vi "TraverseControl_High.vi"(0 "Mode":T3=enum."Read traverse position", 1 "Route Checking?":bool, 2 "Home":T2, 3 "Traverse Name":string, 5 "Extra command String":string, 6 "Work in Tunnel Coordinates":T1, 7 "Model       Roll      Pitch       Yaw (deg)":sgl[](array[numeric]) format="%#.2f", 9 "Final iteration of 3D_Trav Loop":bool=TRUE, 11 "Position input XYZ Always Tunnel":sgl[](array[numeric])=[0.0, 0.0, 0.0] format="%.2f", 12 "Last Part of Move?":bool, 13 "Speed Factor":sgl=1.0 min=0.1 max=5 format="%.2f", 14 "Backlash Compensation?":bool=TRUE) -> (4 "Position Output XYZ":sgl[](array[numeric]) format="%.2f", 10 "Position Correct":bool, 15 "Error String":string)   [LabVIEW 2022 SP3]
uses:
  Anemometry/Anemometry Sub Vis/Gen Trav/Trav_mode.ctl
  Anemometry/Anemometry Sub Vis/Controls/Home.ctl
  Anemometry/Anemometry Sub Vis/Controls/Tunnel_Coordinates.ctl
  Anemometry/Anemometry Sub Vis/Globals/Extra_Commands_Global.vi
  Anemometry/Anemometry Sub Vis/Globals/Trav_pos_global.vi
  Anemometry/Anemometry Sub Vis/Gen Trav/Route mapping/Route_mapping_global.vi
panel:
  out "Offset Array":sgl[](array[numeric])
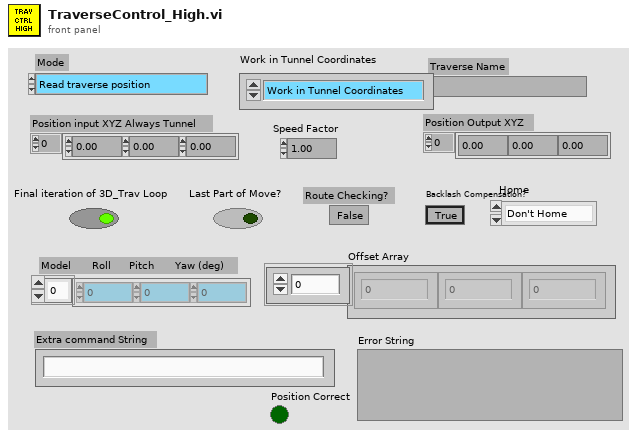
[diagram p1: front panel]
types:
  T1 = typedef "Tunnel_Coordinates.ctl" = enum16{"Work in Tunnel Coordinates", "Work in Model Coordinates"}
  T2 = typedef "Home.ctl" = enum16{"Don't Home", "Home  +X", "Home  -X", "Home  +Y", "Home  -Y", "Home  +Z", "Home  -Z"}
  T3 = typedef "Trav_mode.ctl" = enum16{"Move traverse", "Read traverse position", "Teach Position"}
  T4 = enum16{"To Traverse Coordinates", "To User Coordinates"}
  T5 = typedef "Axis.ctl" = enum16{"X Axis", "X Axis -ve", "Y Axis", "Y Axis -ve", "Z Axis", "Z Axis -ve"}
  T6 = typedef "Box_size.ctl" = cluster{"Max":sgl, "Min":sgl}[]
  T7 = typedef "Exclude_cluster.ctl" = cluster{"Sizes":T6, "Name":string, "Exclude Type":T8}
  T8 = typedef "Exclusion_type.ctl" = enum16{"Exclude completely", "Allow only vertical moves"}
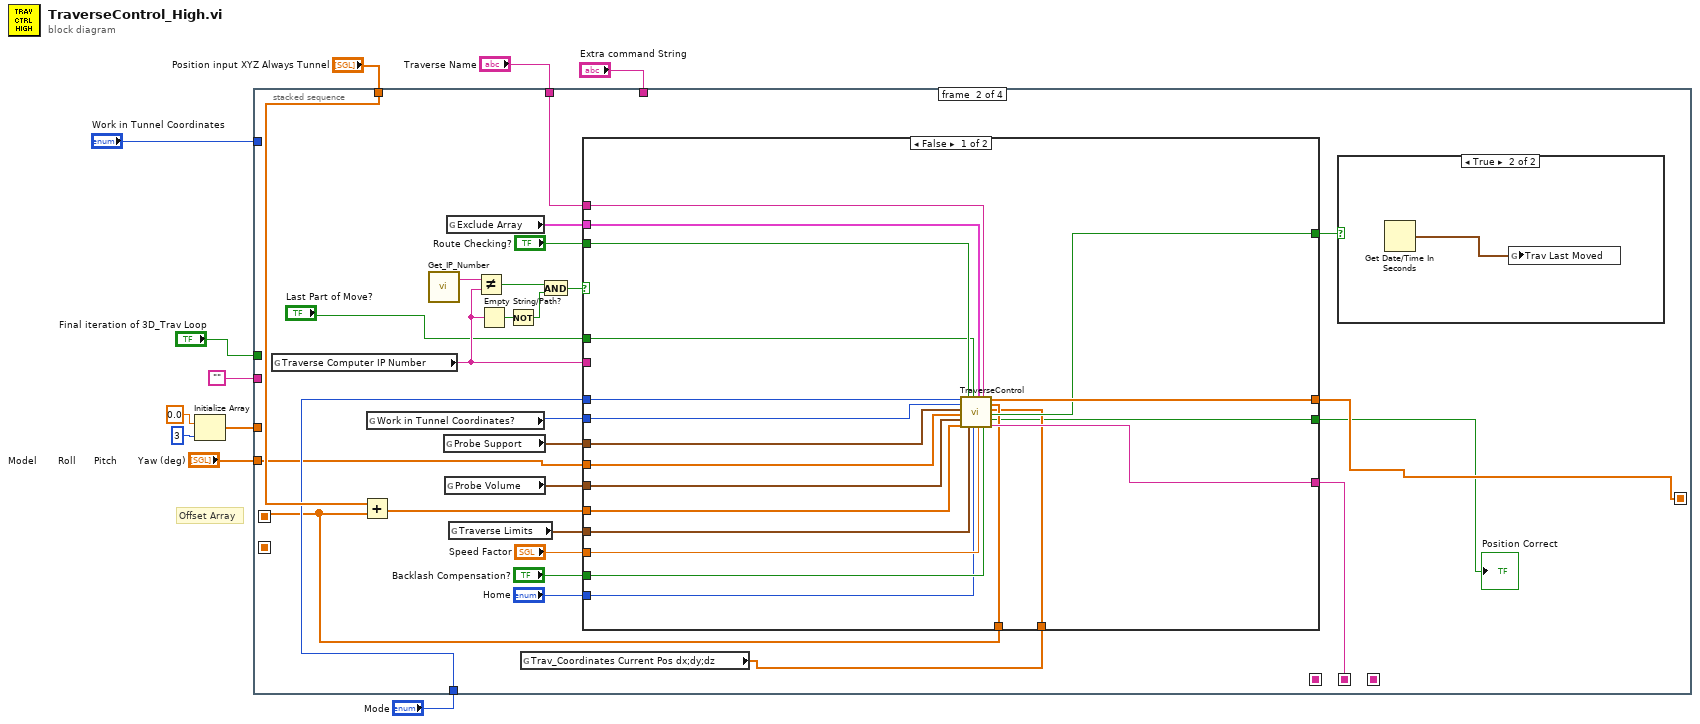
[diagram p0: block diagram]
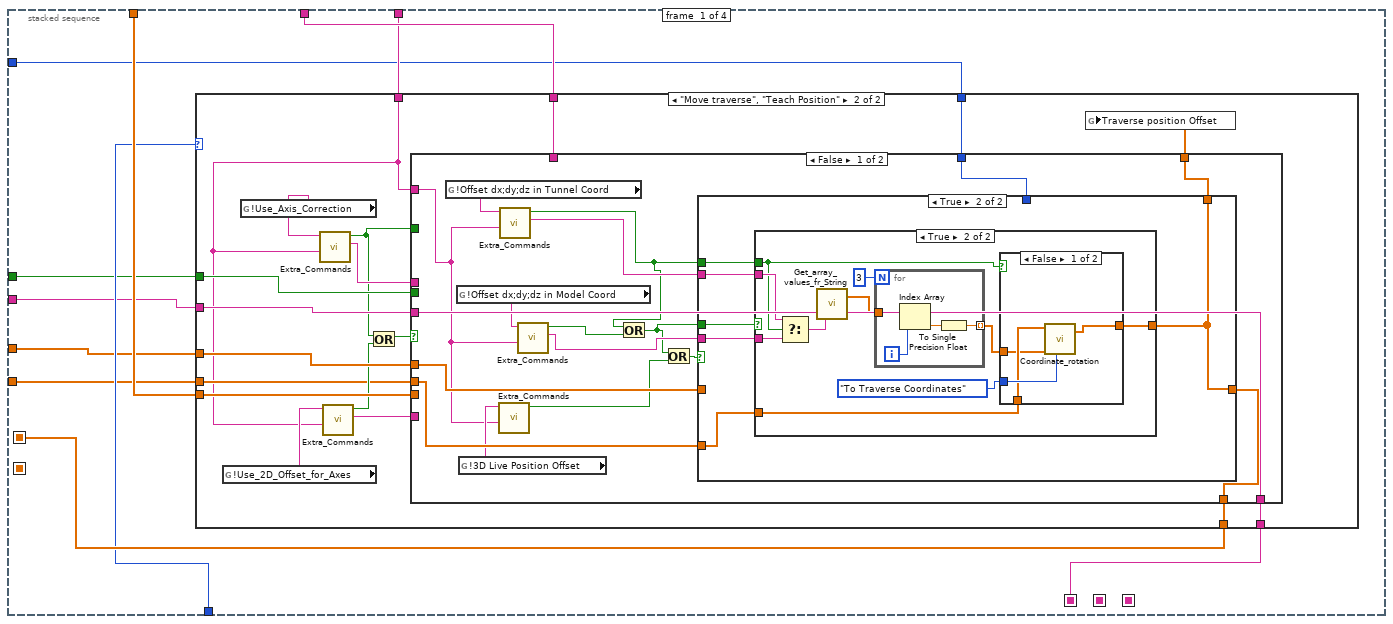
[diagram p2: hidden frame]
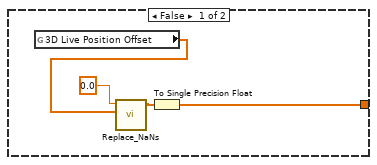
[diagram p5: hidden frame]
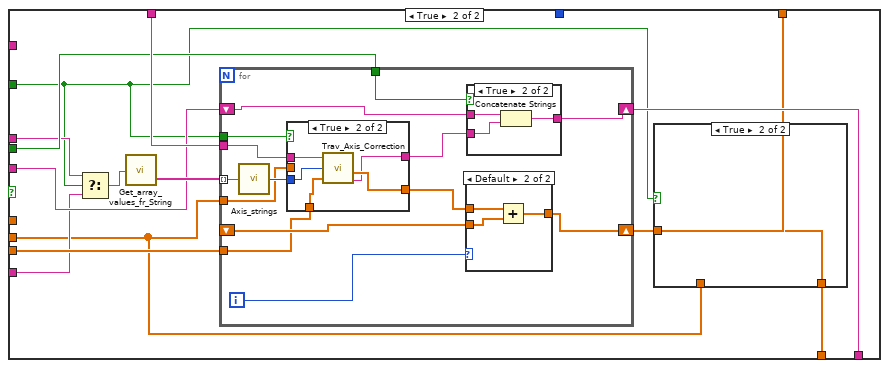
[diagram p7: hidden frame]
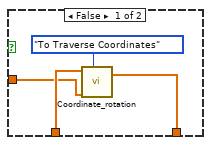
[diagram p8: hidden frame]
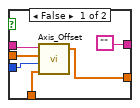
[diagram p9: hidden frame]
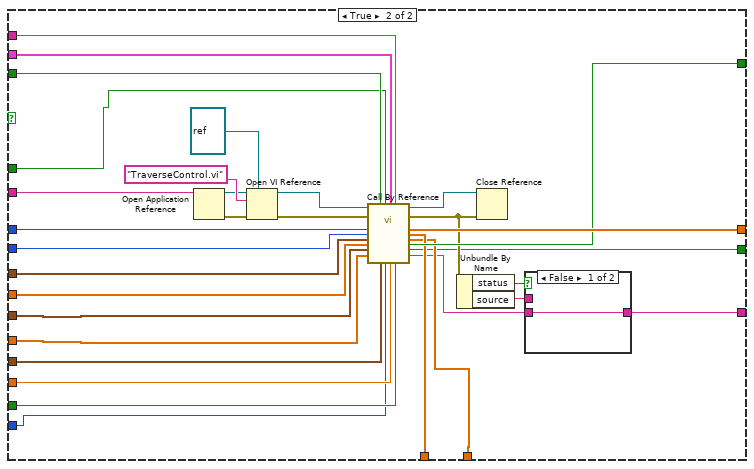
[diagram p13: hidden frame]
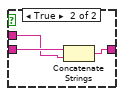
[diagram p14: hidden frame]
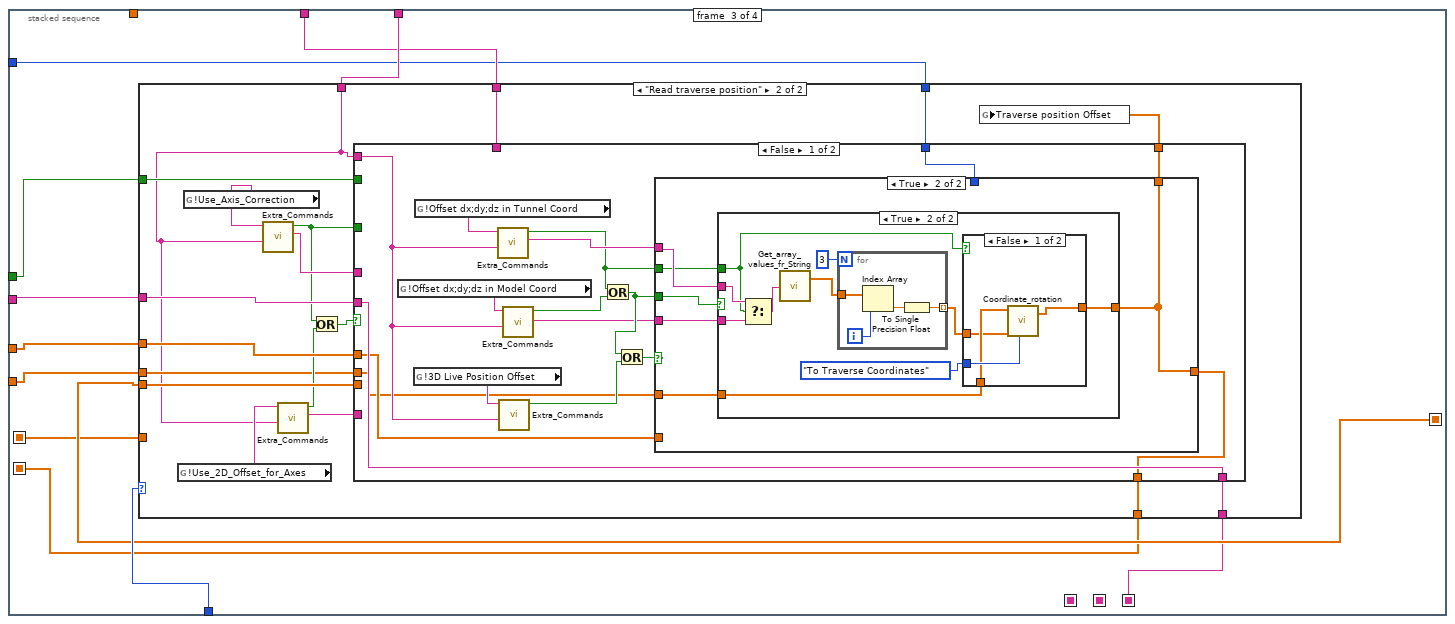
[diagram p15: hidden frame]
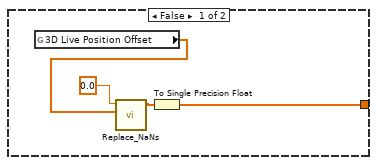
[diagram p18: hidden frame]
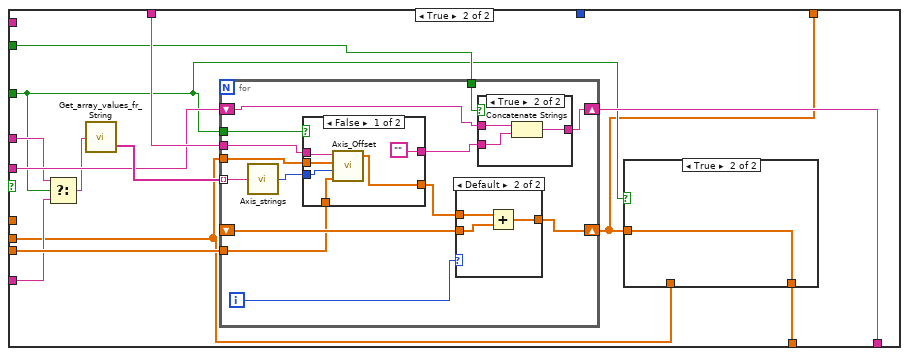
[diagram p20: hidden frame]
diagram:
  # "Offset Array"
  n1 = Initialize Array(sgl 0.0, 3 ("dimension size")) -> (w5:sgl[])
  n2 = stacked-sequence {
    seq-local: [_ w151 _ _] -> [_ _ w232 w360]
    seq-local: [w22 _ _ _] -> [_ w143 w228 _]
    seq-local: [w19 _ _ _] -> [_ _ _ w356]
    seq-local: [_ _ w230 _] -> [_ _ _ w355]
    seq-local: [_ _ w229 _] -> [_ _ _ w358]
    seq-local: [_ w146 _ _] -> [_ _ _ w357]
    tunnel: "Traverse Name" -> [w21 w150 w234 _]
    tunnel: "Position input XYZ Always Tunnel" -> [w20 w149 _ _]
    tunnel: "Mode" -> [w17 w147 w236 _]
    tunnel: "Extra command String" -> [w18 _ w235 _]
    tunnel: w5 -> [w16 _ w231 _]
    tunnel: "" -> [w15 _ w233 _]
    tunnel: "Final iteration of 3D_Trav Loop" -> [w14 _ w227 _]
    tunnel: "Model       Roll      Pitch       Yaw (deg)" -> [w13 w144 w226 _]
    tunnel: "Work in Tunnel Coordinates" -> [w12 _ w225 _]
    frame #0 {
      n3 = case shown="\"Move traverse\", \"Teach Position\"" w17 {
        tunnel: [w23 w41] -> w22
        tunnel: w21 -> [_ w40]
        tunnel: w20 -> [_ w38]
        tunnel: [w24 w37] -> w19
        tunnel: w18 -> [_ w27]
        tunnel: w16 -> [w23 w36]
        tunnel: w15 -> [w24 w35]
        tunnel: w14 -> [_ w34]
        tunnel: w13 -> [_ w28]
        tunnel: w12 -> [_ w25]
        frame Default {
        }
        frame "Move traverse", "Teach Position" {
          n4 = global read "Extra_Commands_Global.vi" "!Use_2D_Offset_for_Axes"() -> (w33:string)
          n5 = global read "Extra_Commands_Global.vi" "!Use_Axis_Correction"() -> (w42:string)
          n6 = call "Extra_Commands.vi"("String to Search"=w27, "Command"=w42) -> ("String Value"=w39:string, "Command Found"=w30:bool)  [unwired: 1 in, 3 out]
          n7 = call "Extra_Commands.vi"("String to Search"=w27, "Command"=w33) -> ("String Value"=w29:string, "Command Found"=w32:bool)  [unwired: 1 in, 3 out]
          n8 = Or(x=w30, y=w32) -> (x .or. y?=w31:bool)
          n9 = case shown="False" w31 {
            tunnel: [w55 w92] -> w41
            tunnel: w38 -> [_ w100]
            tunnel: w40 -> [_ w101]
            tunnel: w39 -> [_ w96]
            tunnel: [w59 w97] -> w37
            tunnel: w35 -> [w59 w99]
            tunnel: w36 -> [w56 _]
            tunnel: w34 -> [_ w98]
            tunnel: w30 -> [_ w91]
            tunnel: w29 -> [_ w95]
            tunnel: w28 -> [w53 w93]
            tunnel: w27 -> [w45 _]
            tunnel: [w52 w90] -> w26
            tunnel: w25 -> [w54 _]
            frame False {
              n10 = global read "Extra_Commands_Global.vi" "!Offset dx;dy;dz in Tunnel Coord"() -> (w58:string)
              n11 = global read "Extra_Commands_Global.vi" "!Offset dx;dy;dz in Model Coord"() -> (w46:string)
              n12 = global read "Extra_Commands_Global.vi" "!3D Live Position Offset"() -> (w49:string)
              n13 = call "Extra_Commands.vi"("String to Search"=w45, "Command"=w49) -> ("Command Found"=w51:bool)  [unwired: 1 in, 4 out]
              n14 = call "Extra_Commands.vi"("String to Search"=w45, "Command"=w58) -> ("String Value"=w57:string, "Command Found"=w48:bool)  [unwired: 1 in, 3 out]
              n15 = call "Extra_Commands.vi"("String to Search"=w45, "Command"=w46) -> ("String Value"=w44:string, "Command Found"=w47:bool)  [unwired: 1 in, 3 out]
              n16 = Or(x=w48, y=w47) -> (x .or. y?=w43:bool)
              n17 = Or(x=w43, y=w51) -> (x .or. y?=w50:bool)
              n18 = case shown="True" w50 {
                tunnel: w57 -> [_ w64]
                tunnel: [w60 w66] -> w55
                tunnel: w56 -> [w60 _]
                tunnel: w54 -> [_ _]
                tunnel: w53 -> [_ w65]
                tunnel: [w60 w66] -> w52
                tunnel: w48 -> [_ w61]
                tunnel: w44 -> [_ w63]
                tunnel: w43 -> [_ w62]
                frame False {
                }
                frame True {
                  n19 = case shown="True" w62 {
                    tunnel: [w67 w75] -> w66
                    tunnel: w65 -> [_ w77]
                    tunnel: w64 -> [_ w74]
                    tunnel: w63 -> [_ w73]
                    tunnel: w61 -> [_ w72]
                    frame False {
                      n20 = global read "Trav_pos_global.vi" "3D Live Position Offset"() -> (w69:sgl[])
                      n21 = call "Replace_NaNs.vi"("Array"=w69, "Replacement"=0.0) -> ("Array Out"=w68:dbl[])  [unwired: 9 in]
                      n22 = To Single Precision Float(number=w68) -> (single precision float=w67:sgl[])
                    }
                    frame True {
                      n23 = Select(t=w74, s=w72, f=w73) -> (s? t:f=w71:string)
                      n24 = call "Get_array_values_fr_String.vi"("String Value"=w71) -> ("Numeric Array"=w79:dbl[])  [unwired: 1 out]
                      n25 = for {
                        N: 3 -> [_]
                        tunnel: w79 -> [w89]
                        tunnel: [w86] -> w76 mode=indexing
                        i -> [w88]
                        n26 = Index Array(array=w89, index=w88) -> (element=w87:dbl)
                        n27 = To Single Precision Float(number=w87) -> (single precision float=w86:sgl)
                      }
                      n28 = case shown="False" w72 {
                        tunnel: T4."To Traverse Coordinates" ("Mode") -> [w84 _]
                        tunnel: w77 -> [w83 _]
                        tunnel: w76 -> [w82 w85]
                        tunnel: [w81 w85] -> w75
                        frame False {
                          n29 = call "Coordinate_rotation.vi"("Roll-Pitch-Yaw"=w83, "Input Position"=w82, "Mode"=w84) -> ("Output Position"=w81:sgl[])  [unwired: 2 in, 1 out]
                        }
                        frame True {
                        }
                      }
                    }
                  }
                }
              }
            }
            frame True {
              n30 = Select(t=w96, s=w91, f=w95) -> (s? t:f=w94:string)
              n31 = call "Get_array_values_fr_String.vi"("String Value"=w94) -> ("String array"=w102:string[])  [unwired: 1 out]
              n32 = for {
                tunnel: w102 -> [w121] mode=indexing
                tunnel: w101 -> [w114]
                tunnel: w100 -> [w112]
                shift-right: [w119] -> w90
                shift-left: _ -> [w120]
                shift-right: [w116] -> w97
                shift-left: w99 -> [w117]
                tunnel: w98 -> [w115]
                tunnel: w91 -> [w108]
                tunnel: w93 -> [w109]
                i -> [w118]
                n33 = call "Axis_strings.vi"("String"=w121) -> ("Enum"=w113:T5)
                n34 = case shown="True" w108 {
                  tunnel: w114 -> [w126 w132]
                  tunnel: w113 -> [w125 w131]
                  tunnel: w112 -> [w124 w130]
                  tunnel: [w127 w129] -> w111
                  tunnel: ["" w128] -> w110
                  tunnel: w109 -> [w122 _]
                  frame False {
                    n35 = call "Axis_Offset.vi"("Position In"=w124, "Axis"=w125, "Roll-Pitch-Yaw"=w122, "Traverse Name"=w126) -> ("Offset Array"=w127:sgl[])  [unwired: 2 out]
                  }
                  frame True {
                    n36 = call "Trav_Axis_Correction.vi"("Traverse Name"=w132, "Axis"=w131, "Position input XYZ"=w130) -> ("Offset Array"=w129:sgl[], "Error String"=w128:string)  [unwired: 2 out]
                  }
                }
                n37 = case shown="Default" w118 {
                  tunnel: w111 -> [w137 w140]
                  tunnel: w120 -> [_ w139]
                  tunnel: [w137 w138] -> w119
                  frame 0 {
                  }
                  frame Default {
                    n38 = Add(x=w140, y=w139) -> (x+y=w138:sgl[])
                  }
                }
                n39 = case shown="True" w115 {
                  tunnel: w110 -> [_ w136]
                  tunnel: w117 -> [w133 w135]
                  tunnel: [w133 w134] -> w116
                  frame False {
                  }
                  frame True {
                    n40 = Concatenate Strings(w135, w136) -> (w134:string)
                  }
                }
              }
              n41 = case shown="True" w91 {
                tunnel: w90 -> [w103 w107]
                tunnel: w93 -> [w106 _]
                tunnel: [w105 w107] -> w92
                frame False {
                  n42 = call "Coordinate_rotation.vi"("Roll-Pitch-Yaw"=w106, "Input Position"=w103, "Mode"=T4."To Traverse Coordinates") -> ("Output Position"=w105:sgl[])  [unwired: 2 in, 1 out]
                }
                frame True {
                }
              }
            }
          }
          n43 = global write "Trav_pos_global.vi" "Traverse position Offset"(w26) -> ()
        }
      }
    }
    frame #1 {
      n44 = global read "Trav_pos_global.vi" "Traverse Computer IP Number"() -> (w161:string)
      n45 = Add(x=w149, y=w143) -> (x+y=w148:sgl[])
      n46 = global read "Trav_pos_global.vi" "Work in Tunnel Coordinates?"() -> (w155:T1)
      n47 = call "Get_IP_Number.vi"() -> ("IP Number"=w167:string)  [unwired: 1 out]
      n48 = global read "Route_mapping_global.vi" "Probe Support"() -> (w154:T6)
      n49 = global read "Route_mapping_global.vi" "Probe Volume"() -> (w156:T6)
      n50 = global read "Route_mapping_global.vi" "Exclude Array"() -> (w158:T7[])
      n51 = global read "Route_mapping_global.vi" "Traverse Limits"() -> (w157:T6)
      n52 = Not Equal?(x=w167, y=w161) -> (x != y?=w160:bool)
      n53 = Empty String/Path?(string/path=w161) -> (empty?=w163:bool)
      n54 = Not(x=w163) -> (.not. x?=w162:bool)
      n55 = global read "Trav_pos_global.vi" "Trav_Coordinates Current Pos dx;dy;dz"() -> (w142:sgl[])
      n56 = And(x=w160, y=w162) -> (x .and. y?=w159:bool)
      n57 = case shown="False" w159 {
        tunnel: "Route Checking?" -> [w181 w220]
        tunnel: w150 -> [w180 w219]
        tunnel: [w187 w218] -> w151
        tunnel: [w188 w210] -> w146
        tunnel: "Backlash Compensation?" -> [w184 w217]
        tunnel: "Speed Factor" -> [w183 w216]
        tunnel: w148 -> [w186 w215]
        tunnel: w144 -> [w185 w214]
        tunnel: w147 -> [w182 w213]
        tunnel: w161 -> [_ w212]
        tunnel: w158 -> [w179 w211]
        tunnel: w157 -> [w178 w207]
        tunnel: w156 -> [w177 w208]
        tunnel: w155 -> [w176 w209]
        tunnel: w154 -> [w175 w206]
        tunnel: "Last Part of Move?" -> [w174 w205]
        tunnel: "Home" -> [w173 w204]
        tunnel: [w172 w203] -> w152
        tunnel: w143 -> [w171 w202]
        tunnel: w142 -> [w170 w201]
        tunnel: [w169 w189] -> w141
        frame False {
          n58 = call "TraverseControl.vi"("Mode"=w182, "Work in Tunnel Coordinates?"=w176, "Probe Support"=w175, "Model       Roll      Pitch       Yaw (deg)"=w185, "Probe Volume"=w177, "Position input XYZ"=w186, "Route Checking?"=w181, "Entire Space"=w178, "Last Part of Move?"=w174, "Home"=w173, "Exclude Array"=w179, "Speed Factor"=w183, "Traverse Name"=w180, "Backlash Compensation?"=w184, "Trav_Coordinates New Pos dx;dy;dz"=w171, "Trav_Coordinates Current Pos dx;dy;dz"=w170) -> ("Position Output XYZ"=w187:sgl[], "Moved?"=w172:bool, "Position Correct"=w169:bool, "Error String"=w188:string)
        }
        frame True {
          n59 = Open Application Reference(11:w212) -> (0:w194:errorcluster, 3:w195:refnum<vi>)  [unwired: 2 in, 1 out]
          n60 = Open VI Reference(type specifier VI Refnum (for type only)=refnum<vi> refnum ("Scout Server"), application reference (local)=w195, vi path="TraverseControl.vi", error in (no error)=w194) -> (vi reference=w198:refnum<vi>, error out=w197:errorcluster)  [unwired: 2 out]
          n61 = call-by-ref "?"(reference=w198, error in=w197, "Mode"=w213, "Work in Tunnel Coordinates?"=w209, "Probe Support"=w206, "Model       Roll      Pitch       Yaw (deg)"=w214, "Probe Volume"=w208, "Position input XYZ"=w215, "Route Checking?"=w220, "Entire Space"=w207, "Last Part of Move?"=w205, "Home"=w204, "Exclude Array"=w211, "Speed Factor"=w216, "Traverse Name"=w219, "Backlash Compensation?"=w217, "Trav_Coordinates New Pos dx;dy;dz"=w202, "Trav_Coordinates Current Pos dx;dy;dz"=w201) -> (reference out=w196:refnum<vi>, error out=w193:errorcluster, "Position Output XYZ"=w218:sgl[], "Moved?"=w203:bool, "Position Correct"=w189:bool, "Error String"=w191:string)
          n62 = Unbundle By Name(w193) -> ("status"=w192:bool, "source"=w190:string)
          n63 = Close Reference(reference=w196, error in (no error)=w193) -> ()  [unwired: 1 out]
          n64 = case shown="False" w192 {
            tunnel: [w221 w224] -> w210
            tunnel: w191 -> [w221 w223]
            tunnel: w190 -> [_ w222]
            frame False {
            }
            frame True {
              n65 = Concatenate Strings(w223, w222) -> (w224:string)
            }
          }
        }
      }
      "Position Correct" <- w141
      n66 = case shown="True" w152 {
        frame False {
        }
        frame True {
          n67 = Get Date/Time In Seconds() -> (seconds since 1Jan1904=w168:timestamp)
          n68 = global write "Trav_pos_global.vi" "Trav Last Moved"(w168) -> ()
        }
      }
    }
    frame #2 {
      n69 = case shown="\"Read traverse position\"" w236 {
        tunnel: [w237 w255] -> w230
        tunnel: w234 -> [_ w254]
        tunnel: w232 -> [_ w252]
        tunnel: [w238 w251] -> w229
        tunnel: w235 -> [_ w241]
        tunnel: w231 -> [_ w250]
        tunnel: w233 -> [w238 w249]
        tunnel: w228 -> [w237 _]
        tunnel: w227 -> [_ w248]
        tunnel: w226 -> [_ w242]
        tunnel: w225 -> [_ w239]
        frame Default {
        }
        frame "Read traverse position" {
          n70 = global read "Extra_Commands_Global.vi" "!Use_2D_Offset_for_Axes"() -> (w247:string)
          n71 = global read "Extra_Commands_Global.vi" "!Use_Axis_Correction"() -> (w256:string)
          n72 = call "Extra_Commands.vi"("String to Search"=w241, "Command"=w256) -> ("String Value"=w253:string, "Command Found"=w244:bool)  [unwired: 1 in, 3 out]
          n73 = call "Extra_Commands.vi"("String to Search"=w241, "Command"=w247) -> ("String Value"=w243:string, "Command Found"=w245:bool)  [unwired: 1 in, 3 out]
          n74 = Or(x=w244, y=w245) -> (x .or. y?=w246:bool)
          n75 = case shown="False" w246 {
            tunnel: [w267 w307] -> w255
            tunnel: w252 -> [_ w314]
            tunnel: w254 -> [_ w315]
            tunnel: w253 -> [_ w310]
            tunnel: [w272 w313] -> w251
            tunnel: w249 -> [w272 w312]
            tunnel: w250 -> [w270 _]
            tunnel: w248 -> [_ w311]
            tunnel: w244 -> [_ w305]
            tunnel: w243 -> [_ w309]
            tunnel: w242 -> [w257 w306]
            tunnel: w241 -> [w262 _]
            tunnel: [w268 w304] -> w240
            tunnel: w239 -> [w269 _]
            frame False {
              n76 = global read "Extra_Commands_Global.vi" "!Offset dx;dy;dz in Model Coord"() -> (w263:string)
              n77 = global read "Extra_Commands_Global.vi" "!3D Live Position Offset"() -> (w266:string)
              n78 = global read "Extra_Commands_Global.vi" "!Offset dx;dy;dz in Tunnel Coord"() -> (w273:string)
              n79 = call "Extra_Commands.vi"("String to Search"=w262, "Command"=w273) -> ("String Value"=w271:string, "Command Found"=w259:bool)  [unwired: 1 in, 3 out]
              n80 = call "Extra_Commands.vi"("String to Search"=w262, "Command"=w266) -> ("Command Found"=w264:bool)  [unwired: 1 in, 4 out]
              n81 = call "Extra_Commands.vi"("String to Search"=w262, "Command"=w263) -> ("String Value"=w258:string, "Command Found"=w260:bool)  [unwired: 1 in, 3 out]
              n82 = Or(x=w259, y=w260) -> (x .or. y?=w261:bool)
              n83 = Or(x=w261, y=w264) -> (x .or. y?=w265:bool)
              n84 = case shown="True" w265 {
                tunnel: [w274 w280] -> w267
                tunnel: w270 -> [w274 _]
                tunnel: w269 -> [_ _]
                tunnel: [w274 w280] -> w268
                tunnel: w271 -> [_ w279]
                tunnel: w261 -> [_ w278]
                tunnel: w259 -> [_ w277]
                tunnel: w258 -> [_ w276]
                tunnel: w257 -> [_ w275]
                frame False {
                }
                frame True {
                  n85 = case shown="True" w278 {
                    tunnel: [w281 w285] -> w280
                    tunnel: w279 -> [_ w292]
                    tunnel: w277 -> [_ w289]
                    tunnel: w276 -> [_ w291]
                    tunnel: w275 -> [_ w287]
                    frame False {
                      n86 = global read "Trav_pos_global.vi" "3D Live Position Offset"() -> (w283:sgl[])
                      n87 = call "Replace_NaNs.vi"("Array"=w283, "Replacement"=0.0) -> ("Array Out"=w282:dbl[])  [unwired: 9 in]
                      n88 = To Single Precision Float(number=w282) -> (single precision float=w281:sgl[])
                    }
                    frame True {
                      n89 = Select(t=w292, s=w289, f=w291) -> (s? t:f=w290:string)
                      n90 = call "Get_array_values_fr_String.vi"("String Value"=w290) -> ("Numeric Array"=w293:dbl[])  [unwired: 1 out]
                      n91 = for {
                        N: 3 -> [_]
                        tunnel: w293 -> [w303]
                        tunnel: [w300] -> w286 mode=indexing
                        i -> [w302]
                        n92 = Index Array(array=w303, index=w302) -> (element=w301:dbl)
                        n93 = To Single Precision Float(number=w301) -> (single precision float=w300:sgl)
                      }
                      n94 = case shown="False" w289 {
                        tunnel: T4."To Traverse Coordinates" ("Mode") -> [w298 _]
                        tunnel: w287 -> [w297 _]
                        tunnel: w286 -> [w296 w299]
                        tunnel: [w295 w299] -> w285
                        frame False {
                          n95 = call "Coordinate_rotation.vi"("Roll-Pitch-Yaw"=w297, "Input Position"=w296, "Mode"=w298) -> ("Output Position"=w295:sgl[])  [unwired: 2 in, 1 out]
                        }
                        frame True {
                        }
                      }
                    }
                  }
                }
              }
            }
            frame True {
              n96 = Select(t=w310, s=w305, f=w309) -> (s? t:f=w308:string)
              n97 = call "Get_array_values_fr_String.vi"("String Value"=w308) -> ("String array"=w316:string[])  [unwired: 1 out]
              n98 = for {
                tunnel: w316 -> [w335] mode=indexing
                tunnel: w315 -> [w324]
                tunnel: w314 -> [w326]
                shift-right: [w333] -> w304
                shift-left: _ -> [w334]
                shift-right: [w330] -> w313
                shift-left: w312 -> [w331]
                tunnel: w311 -> [w329]
                tunnel: w305 -> [w323]
                tunnel: w306 -> [w322]
                i -> [w332]
                n99 = call "Axis_strings.vi"("String"=w335) -> ("Enum"=w325:T5)
                n100 = case shown="False" w323 {
                  tunnel: w324 -> [w340 w346]
                  tunnel: w325 -> [w339 w345]
                  tunnel: w326 -> [w338 w344]
                  tunnel: [w341 w343] -> w327
                  tunnel: ["" w342] -> w328
                  tunnel: w322 -> [w336 _]
                  frame False {
                    n101 = call "Axis_Offset.vi"("Position In"=w338, "Axis"=w339, "Roll-Pitch-Yaw"=w336, "Traverse Name"=w340) -> ("Offset Array"=w341:sgl[])  [unwired: 2 out]
                  }
                  frame True {
                    n102 = call "Trav_Axis_Correction.vi"("Traverse Name"=w346, "Axis"=w345, "Position input XYZ"=w344) -> ("Offset Array"=w343:sgl[], "Error String"=w342:string)  [unwired: 2 out]
                  }
                }
                n103 = case shown="Default" w332 {
                  tunnel: w327 -> [w351 w354]
                  tunnel: w334 -> [_ w353]
                  tunnel: [w351 w352] -> w333
                  frame 0 {
                  }
                  frame Default {
                    n104 = Add(x=w354, y=w353) -> (x+y=w352:sgl[])
                  }
                }
                n105 = case shown="True" w329 {
                  tunnel: w328 -> [_ w350]
                  tunnel: w331 -> [w347 w349]
                  tunnel: [w347 w348] -> w330
                  frame False {
                  }
                  frame True {
                    n106 = Concatenate Strings(w349, w350) -> (w348:string)
                  }
                }
              }
              n107 = case shown="True" w305 {
                tunnel: w304 -> [w320 w321]
                tunnel: w306 -> [w319 _]
                tunnel: [w318 w321] -> w307
                frame False {
                  n108 = call "Coordinate_rotation.vi"("Roll-Pitch-Yaw"=w319, "Input Position"=w320, "Mode"=T4."To Traverse Coordinates") -> ("Output Position"=w318:sgl[])  [unwired: 2 in, 1 out]
                }
                frame True {
                }
              }
            }
          }
          n109 = global write "Trav_pos_global.vi" "Traverse position Offset"(w240) -> ()
        }
      }
    }
    frame #3 {
      n110 = global write "Trav_pos_global.vi" "Trav_Coordinates Current Pos dx;dy;dz"(w355) -> ()
      n111 = Subtract(x=w360, y=w355) -> (x-y=→"Position Output XYZ":sgl[])
      n112 = Concatenate Strings(w356, w357, w358) -> (→"Error String":string)
      "Offset Array" <- w355
    }
  }
